vi "Test Login.vi"   [LabVIEW 2020]
uses:
  [V] Login/[V] Login/[V] Login.lvclass
  C:/Program Files (x86)/National Instruments/LabVIEW 2020/vi.lib/ActorFramework/Actor/Actor.lvclass
  [V] Login/[V] Login/[V] Login.lvclass/[V] Login.ctl
  [V] Login/[V] Login/Accessor/Write Ring Picture Path.vi
  <vilib>/ActorFramework/Actor/Actor.lvclass
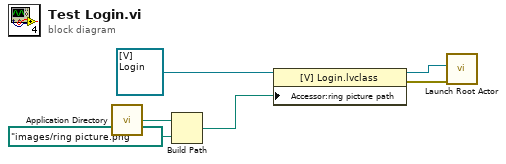
[diagram p0: block diagram]
diagram:
  n1 = call <vilib>:"Application Directory.vi"() -> ("Application Directory"=w5:path)
  n2 = Build Path(base path=w5, name or relative path=path "images/ring picture.png") -> (appended path=w3:path)
  n3 = property class="[V] Login.lvclass"(reference=refnum<class "[V] Login.lvclass"> refnum ("[V] Login.lvlib:[V] Login.lvclass"), "Accessor:ring picture path"=w3) -> (reference out=w1:refnum<class "[V] Login.lvclass">, error out=w2:errorcluster)  [unwired: 1 in]
  n4 = call <vilib>:"Launch Root Actor.vi"("error in (no error)"=w2, "Actor"=w1) -> ()  [unwired: 8 in, 2 out]
